vi "Global 1.vi"() -> ()   [LabVIEW 2019]
panel:
  out "right dwon":i32
  out "right center":i32
  out "right top":i32
  out "center down":i32
  out "center middel":i32
  out "center top":i32
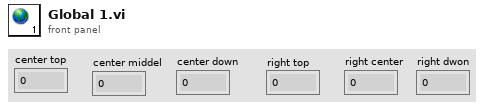
[diagram p1: front panel]
diagram:
